vi "call dll with path.vi"() -> ()   [LabVIEW 2020]
panel:
  out "deleted path":path
  in  "text":string
  out "dll exit":bool
  out "error out 2":errorcluster
  in  "stop":bool
  out "base_path":string="C:\\Users\\duyga\\OneDrive\\??????\\WORKS\\Nissan GPS\\gps-sdr-sim-dll - add base path"
  out "error out":errorcluster
  in  "param":string="-e brdc0010.22n -u circle.csv -d 10 -o filename"
  out "return code":i32
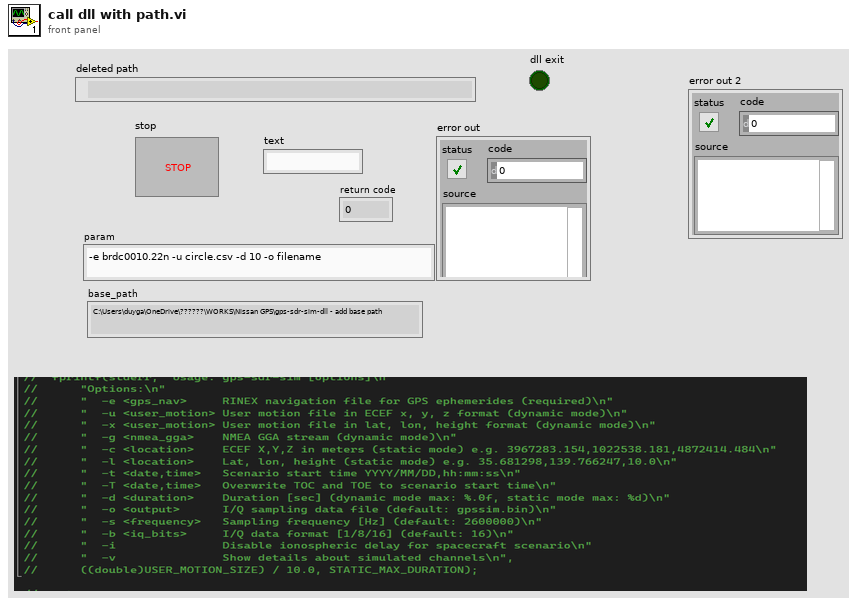
[diagram p1: front panel]
types:
  T1 = enum16{"open", "replace", "create", "open or create", "replace or create", "replace or create with confirmation"}
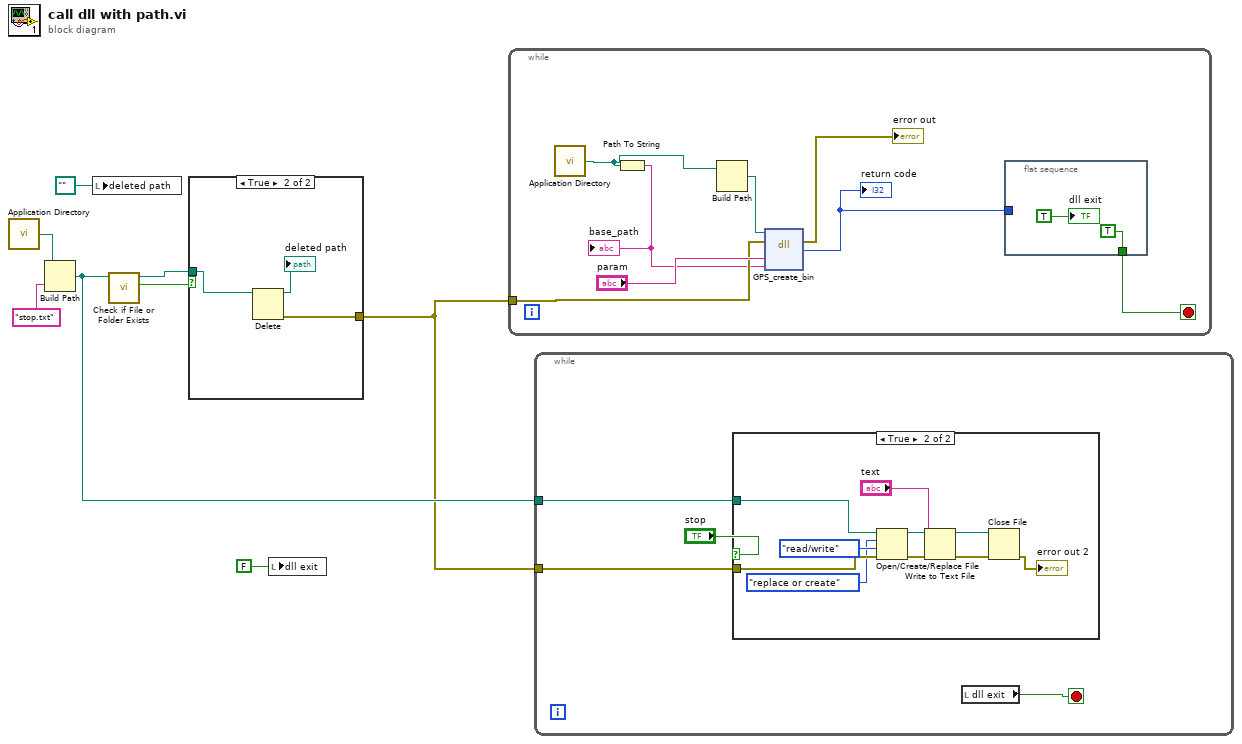
[diagram p0: block diagram]
diagram:
  n1 = call <vilib>:"Application Directory.vi"() -> ("Application Directory"=w8:path)
  n2 = Build Path(base path=w8, name or relative path="stop.txt") -> (appended path=w5:path)
  n3 = local write "deleted path"(path "" ("deleted path")) -> ()
  n4 = call <vilib>:"Check if File or Folder Exists.vi"("path"=w5) -> ("file or folder exists?"=w4:bool, "dup path"=w3:path)  [unwired: 8 in, 1 out]
  n5 = case shown="True" w4 {
    tunnel: w3 -> [_ w11]
    tunnel: [_ w10] -> w2
    frame False {
    }
    frame True {
      n6 = Delete(path (use dialog)=w11) -> (deleted path=→"deleted path":path, error out=w10:errorcluster)  [unwired: 4 in, 1 out]
    }
  }
  n7 = local write "dll exit"(FALSE ("dll exit")) -> ()
  n8 = while {
    tunnel: w2 -> [w16]
    stop <- w17 stop-if-true
    n9 = call <vilib>:"Application Directory.vi"() -> ("Application Directory"=w14:path)
    n10 = Path To String(path=w14) -> (string=w15:string)
    "base_path" <- w15
    n11 = Build Path(base path=w14) -> (name or relative path=w12:path, appended path=w13:path)
    n12 = dll-call lib="PTH2iabs CUsersduygaOneDriveデスクトップWORKS\nNissan GPS\tbuild dllGPS_SIM_CREATE_BIN.dll" fn="GPS_create_bin"(path in=w13, error in=w16, "param"="param", "base_path"=w15) -> (error out=→"error out":errorcluster, "return code"=w18:i32)  [unwired: 3 in, 1 out]
    "return code" <- w18
    n13 = flat-sequence {
      tunnel: w18 -> [_]
      tunnel: [TRUE] -> w17
      frame #0 {
        "dll exit" <- TRUE ("dll exit")
      }
    }
  }
  n14 = while {
    tunnel: w2 -> [w26]
    tunnel: w5 -> [w25]
    stop <- w24 stop-if-true
    n15 = case shown="True" "stop" {
      tunnel: w25 -> [_ w32]
      tunnel: w26 -> [_ w31]
      frame False {
      }
      frame True {
        n16 = Open/Create/Replace File(file path (use dialog)=w32, error in=w31, operation (0:open)=T1."replace or create", access (0:read/write)=enum16{"read/write", "read-only", "write-only"}."read/write") -> (refnum out=w27:refnum<file>, error out=w30:errorcluster)  [unwired: 2 in, 1 out]
        n17 = Write to Text File(file (use dialog)=w27, text="text", error in=w30) -> (refnum out=w33:refnum<file>, error out=w34:errorcluster)  [unwired: 1 in, 1 out]
        n18 = Close File(refnum=w33, error in=w34) -> (error out=→"error out 2":errorcluster)  [unwired: 1 out]
      }
    }
    n19 = local read "dll exit"() -> (w24:bool)
  }
